vi "initData.vi"(8 "error in (no error)":errorcluster) -> (0 "error out":errorcluster)   [LabVIEW 2017, in "programControl.lvlib"]
doc: "This VI initialises the shutdown, enable assistance and error variables to false."
uses:
  programControl.lvlib
  TypeDefs/dataIn.ctl
  TypeDefs/dataOut.ctl
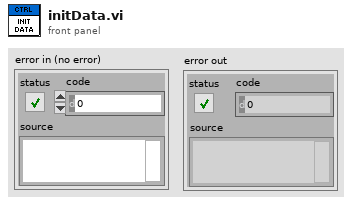
[diagram p1: front panel]
types:
  T1 = typedef "dataOut.ctl" = cluster{"X0pos":dbl, "Y0pos":dbl, "Z0pos":dbl, "Fx":dbl, "Fy":dbl, "Fz":dbl, "Encoder1":i32, "Encoder2":i32, "Pot1":dbl, "Pot2":dbl, "Theta0":dbl, "Theta1":dbl, "X1pos":dbl, "Y1pos":dbl, "Z1pos":dbl, "X2pos":dbl, "Y2pos":dbl, "Z2pos":dbl, "ErrorOccurred":bool}
  T2 = typedef "dataIn.ctl" = cluster{"Xtarget":dbl, "Ytarget":dbl, "Ztarget":dbl, "X_Attractor1":dbl, "Y_Attractor1":dbl, "Z_Attractor1":dbl, "X_Attractor2":dbl, "Y_Attractor2":dbl, "Z_Attractor2":dbl, "Traj_Flag":bool, "DeadZone":dbl, "Assistance":bool, "Shutdown":bool, "AssistanceLevel":dbl}
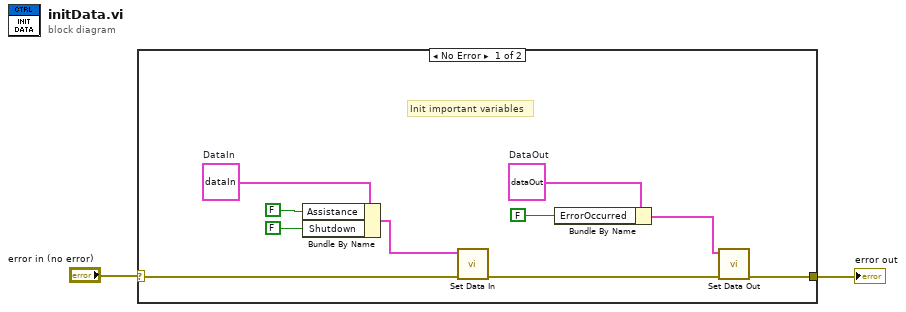
[diagram p0: block diagram]
diagram:
  n1 = case shown="No Error" "error in (no error)" {
    selector: "error in (no error)" -> [w8 w13]
    tunnel: [w5 w13] -> w1
    frame No Error {
      w10 = T1 {"X0pos"=0.0, "Y0pos"=0.0, "Z0pos"=0.0, "Fx"=0.0, "Fy"=0.0, "Fz"=0.0, "Encoder1"=0, "Encoder2"=0, "Pot1"=0.0, "Pot2"=0.0, "Theta0"=0.0, "Theta1"=0.0, "X1pos"=0.0, "Y1pos"=0.0, "Z1pos"=0.0, "X2pos"=0.0, "Y2pos"=0.0, "Z2pos"=0.0, "ErrorOccurred"=FALSE}  # DataOut
      w12 = T2 {"Xtarget"=0.0, "Ytarget"=0.0, "Ztarget"=0.0, "X_Attractor1"=0.0, "Y_Attractor1"=0.0, "Z_Attractor1"=0.0, "X_Attractor2"=0.0, "Y_Attractor2"=0.0, "Z_Attractor2"=0.0, "Traj_Flag"=FALSE, "DeadZone"=0.0, "Assistance"=FALSE, "Shutdown"=FALSE, "AssistanceLevel"=0.0}  # DataIn
      # "Init important variables"
      n2 = Bundle By Name(cluster=w12, "Assistance"=FALSE, "Shutdown"=FALSE) -> (w7:T2)
      n3 = call "Set Data In.vi"("error in (no error)"=w8, "DataIn"=w7) -> ("error out"=w6:errorcluster)  [unwired: 9 in]
      n4 = Bundle By Name(cluster=w10, "ErrorOccurred"=FALSE) -> (w4:T1)
      n5 = call "Set Data Out.vi"("error in (no error)"=w6, "DataOut"=w4) -> ("error out"=w5:errorcluster)  [unwired: 9 in]
    }
    frame Error {
    }
  }
  "error out" <- w1
